vi "byteArrayToI32.vi"(8 "error in (no error)":errorcluster, 9 "StartIndex":i32, 10 "ByteArrayIn":u8[](array[numeric])) -> (0 "error out":errorcluster, 1 "EndIndex":i32, 2 "ByteArrayOut":u8[](array[numeric]), 3 "I32":i32)   [LabVIEW 2013, in "BSON.lvlib"]
uses:
  BSON.lvlib
  status.ctl
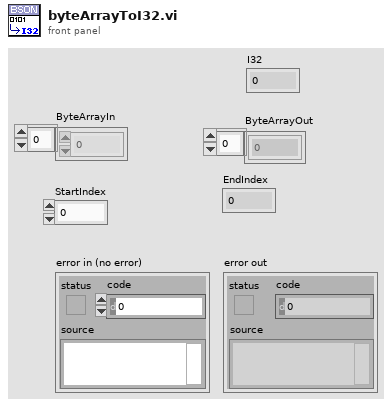
[diagram p1: front panel]
types:
  T1 = typedef "BSON.lvlib/status.ctl" = enum16{"Stream Corrupted or Ended Abruptly", "Incorrect Type In Stream", "ObjectID Invalid", "Method Not Implemented", "Invalid Name", "Invalid URI", "AutoReconnect", "Operation Failed", "Incorrectly Configured", "Cursor Not Found", "Timeout", "Invalid Type", "Empty Name", "Duplicate Name", "MD5Incorrect"}
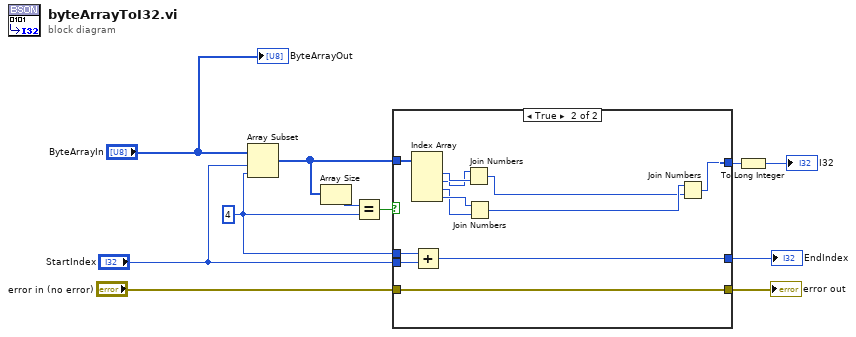
[diagram p0: block diagram]
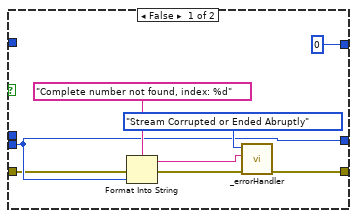
[diagram p2: hidden frame]
diagram:
  w2 = 4 ("y")
  n1 = Array Subset(array="ByteArrayIn", index="StartIndex", length=w2) -> (w4:u8[])
  n2 = Array Size(array=w4) -> (size(s)=w11:i32)
  n3 = Equal?(x=w11, y=w2) -> (x = y?=w10:bool)
  n4 = case shown="True" w10 {
    tunnel: [u32 0 w26] -> w9
    tunnel: "error in (no error)" -> [w13 w25]
    tunnel: [w12 w25] -> w6
    tunnel: w4 -> [_ w24]
    tunnel: "StartIndex" -> [w14 w22]
    tunnel: w2 -> [_ w21]
    tunnel: [w14 w20] -> w1
    frame False {
      n5 = Format Into String(format string="Complete number not found, index: %d" ("Additional Text"), error in=w13, w14) -> (resulting string=w15:string, error out=w16:errorcluster)  [unwired: 1 in]
      n6 = call "_errorHandler.vi"("error in (no error)"=w16, "Additional Text"=w15, "Error Type"=status."Stream Corrupted or Ended Abruptly") -> ("error out"=w12:errorcluster)  [unwired: 8 in]
    }
    frame True {
      n7 = Index Array(array=w24) -> (element #1=w31:u8, element #2=w30:u8, element #3=w23:u8, element #4=w29:u8)  [unwired: 4 in]
      n8 = Add(x=w21, y=w22) -> (x+y=w20:i32)
      n9 = Join Numbers(hi=w30, lo=w31) -> ((hi.lo)=w27:u16)
      n10 = Join Numbers(hi=w29, lo=w23) -> ((hi.lo)=w28:u16)
      n11 = Join Numbers(hi=w28, lo=w27) -> ((hi.lo)=w26:u32)
    }
  }
  "error out" <- w6
  "EndIndex" <- w1
  n12 = To Long Integer(number=w9) -> (32bit integer=→"I32":i32)
  "ByteArrayOut" <- "ByteArrayIn"
